vi "HP Loop.vi"(8 "error in (no error)":errorcluster, 11 "ValveControlModule in":refnum<class "DigitalControlModule.lvclass">) -> (0 "error out":errorcluster, 3 "ValveControlModule out":refnum<class "DigitalControlModule.lvclass">)   [LabVIEW 2023, in "VolatusControl.lvlib" / "DigitalControlModule.lvclass"]
uses:
  DigitalControlModule.lvclass
  DigitalControlModule.lvclass/DigitalControlModule.ctl
  <vilib>/Platform/TimedLoop/XDataNode/wakeup.ctl
  <vilib>/Platform/TimedLoop/XDataNode/XDNodeRunTimeDep.lvlib
  <vilib>/Platform/TimedLoop/XDataNode/nitl_modes.ctl
  <vilib>/Platform/TimedLoop/XDataNode/timing_clust.ctl
  <vilib>/platform/TimedLoop/XDataNode/XDataNode.xnode
  Volatus/Module/Module.lvclass
  C:/dev/volatus/mts-volatus-super/libs/lv-volatus/Volatus/Module/Module.lvclass
  C:/dev/volatus/mts-volatus-super/libs/lv-volatus/VolatusControl/DigitalControlModule/DigitalControlModule.lvclass
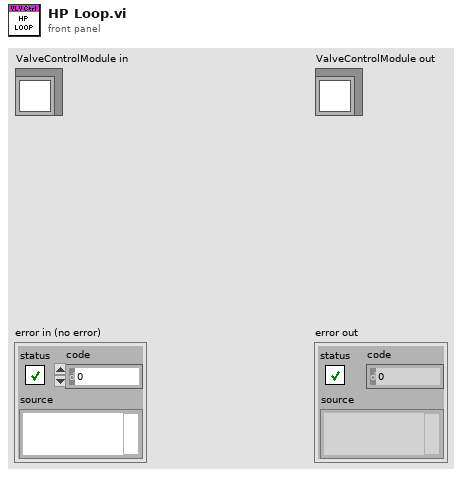
[diagram p1: front panel]
types:
  T1 = typedef "XDNodeRunTimeDep.lvlib/timing_clust.ctl" = cluster{"Expected End [f-1]":u64, "Actual End [f-1]":u64, "Finished Late? [f-1]":bool, "Expected End [i-1]":u64, "Actual End [i-1]":u64, "Finished Late? [i-1]":bool, "Expected Start [i]":u64, "Actual Start [i]":u64, "Expected Start [f]":u64, "Actual Start [f]":u64, "Source Name":string, "Structure Name":string, "Period":i64, "Deadline":i64, "Offset":i64, "Start":i64, "Priority":i32, "Timeout":i32, "Mode":T2, "Wakeup Reason":T3, "Error":errorcluster, "Source Type":string, "Secondary Source Type":string, "Global End Time":u64, "Global Start Time":u64, "Frame Duration":u64, "Iteration Duration":u64, "Assigned CPU":i32, "I/O Scan Engine Mode":u32}
  T2 = typedef "XDNodeRunTimeDep.lvlib/nitl_modes.ctl" = enum32{"No Change", "Process missed periods, maintain original phase", "Discard missed periods, maintain original phase", "Process missed periods, ignore original phase", "Discard missed periods, ignore original phase"}
  T3 = typedef "XDNodeRunTimeDep.lvlib/wakeup.ctl" = enum32{"Normal", "Aborted", "Asynchronous wakeup", "Timing source error", "Timed loop error", "Timeout"}
  T4 = enum32{"Invalid", "Standard", "Closed", "Hidden", "Minimized", "Maximized"}
  T5 = typedef "CmdDigitalMultiple.lvlib/Data.ctl" = cluster{"values":T6[]}
  T6 = typedef "CmdDigital.lvlib/Data.ctl" = cluster{"channel":string, "value":bool}
  T7 = typedef "CmdAnalogMultiple.lvlib/Data.ctl" = cluster{"values":T8[]}
  T8 = typedef "CmdAnalog.lvlib/Data.ctl" = cluster{"channel":string, "value":dbl}
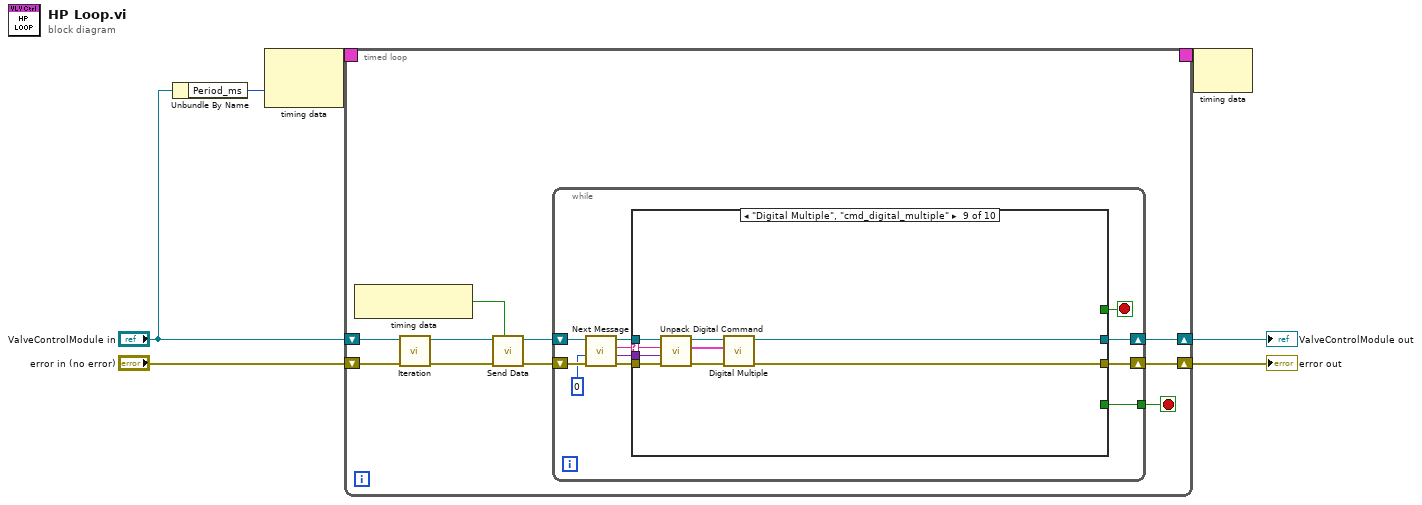
[diagram p0: block diagram]
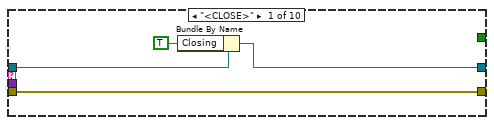
[diagram p2: hidden frame]
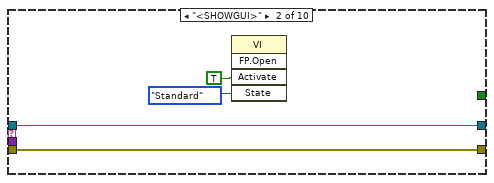
[diagram p3: hidden frame]
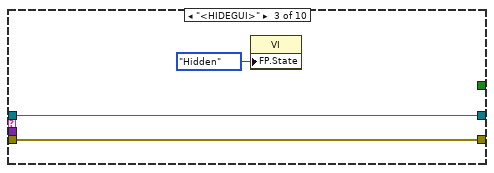
[diagram p4: hidden frame]
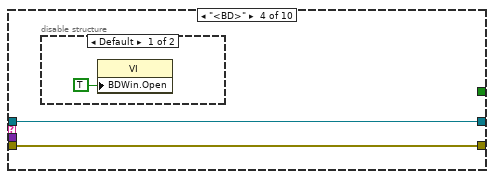
[diagram p5: hidden frame]
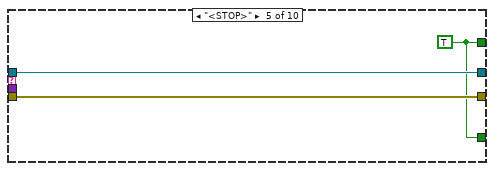
[diagram p7: hidden frame]
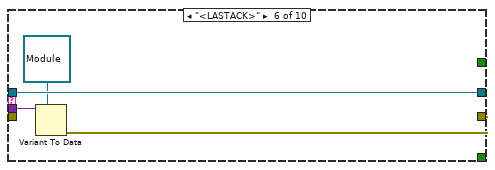
[diagram p8: hidden frame]
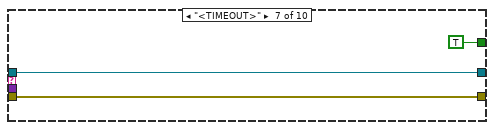
[diagram p9: hidden frame]
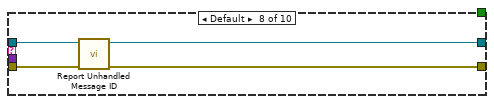
[diagram p10: hidden frame]
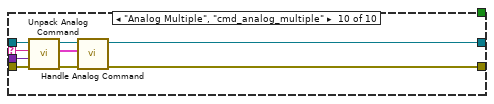
[diagram p11: hidden frame]
diagram:
  n1 = Unbundle By Name("ValveControlModule in") -> ("Period_ms"=w1:i64)
  n2 = node-c288(w1) -> (w7:T1)  [unwired: 1 in]
  n3 = timed-loop {
    shift-right: [w17] -> w4
    shift-left: "ValveControlModule in" -> [w12]
    shift-right: [w16] -> w3
    shift-left: "error in (no error)" -> [w11]
    timing: w7 -> [_]
    timing-out: [_] -> w6
    stop <- w15 stop-if-true
    n4 = node-c288() -> (w8:bool)  [unwired: 1 in]
    n5 = call "Iteration.vi"("error in (no error)"=w11, "ValveControlModule in"=w12) -> ("error out"=w13:errorcluster, "ValveControlModule out"=w14:refnum<class "DigitalControlModule.lvclass">)  [unwired: 8 in]
    n6 = call "Send Data.vi"("Finished Late"=w8, "error in (no error)"=w13, "ValveControlModule in"=w14) -> ("error out"=w10:errorcluster, "ValveControlModule out"=w9:refnum<class "DigitalControlModule.lvclass">)  [unwired: 7 in]
    n7 = while {
      tunnel: [w25] -> w15
      shift-right: [w26] -> w16
      shift-left: w10 -> [w23]
      shift-right: [w27] -> w17
      shift-left: w9 -> [w22]
      stop <- w20 stop-if-true
      n8 = call "Next Message.vi"("error in (no error)"=w23, "Timeout/Period ms (-1)"=0 ("Timeout ms (-1)"), "Module in"=w22) -> ("error out"=w30:errorcluster, "Data"=w24:variant, "ID"=w29:string, "Module out"=w28:refnum<class "DigitalControlModule.lvclass">)  [unwired: 5 in]
      n9 = case shown="\"Digital Multiple\", \"cmd_digital_multiple\"" w29 {
        selector: w29 -> [_ _ _ _ _ _ _ _ w63 w73]
        tunnel: w30 -> [w34 w37 w40 w42 w46 _ w53 w58 w61 w75]
        tunnel: w28 -> [w33 w38 w41 w43 w47 w51 w54 w56 w67 w76]
        tunnel: [w32 w38 w41 w43 w47 w51 w54 w55 w65 w69] -> w27
        tunnel: [w34 w37 w40 w42 w46 w48 w53 w57 w66 w68] -> w26
        tunnel: [_ _ _ _ w45 _ _ _ _ _] -> w25
        tunnel: w24 -> [_ _ _ _ _ w50 _ _ w62 w74]
        tunnel: [_ _ _ _ w45 _ TRUE _ _ _] -> w20
        frame "<CLOSE>" {
          n10 = Bundle By Name(cluster=w33, "Closing"=TRUE) -> (w32:refnum<class "DigitalControlModule.lvclass">)
        }
        frame "<SHOWGUI>" {
          n11 = invoke class="VI" method="FP.Open"("Activate"=TRUE ("Activate?"), "State"=T4."Standard") -> ()  [unwired: 3 in, 5 out]
        }
        frame "<HIDEGUI>" {
          n12 = property class="VI"("FP.State"=T4."Hidden" ("Front Panel Window:State")) -> ()  [unwired: 2 in, 2 out]
        }
        frame "<BD>" {
          n13 = disable-structure shown="Default" {
            frame condition #0 (active) {
              n14 = property class="VI"("BDWin.Open"=TRUE ("Block Diagram Window:Open")) -> ()  [unwired: 2 in, 2 out]
            }
            frame condition #1 {
            }
          }
        }
        frame "<STOP>" {
          w45 = TRUE
        }
        frame "<LASTACK>" {
          n15 = Variant To Data(type=refnum<class "Module.lvclass"> refnum ("Volatus:Module"), Variant=w50) -> (error out=w48:errorcluster)  [unwired: 1 in, 1 out]
        }
        frame "<TIMEOUT>" {
        }
        frame Default {
          n16 = call "Report Unhandled Message ID.vi"("error in (no error)"=w58, "Module in"=w56) -> ("error out"=w57:errorcluster, "Module out"=w55:refnum<class "DigitalControlModule.lvclass">)  [unwired: 8 in]
        }
        frame "Digital Multiple", "cmd_digital_multiple" {
          n17 = call "Unpack Digital Command.vi"("error in (no error)"=w61, "Data"=w62, "Type"=w63, "Module in"=w67) -> ("error out"=w60:errorcluster, "CmdDigitalMultiple"=w59:T5, "Module out"=w64:refnum<class "DigitalControlModule.lvclass">)  [unwired: 3 in, 2 out]
          n18 = call "Digital Multiple.vi"("error in (no error)"=w60, "Data"=w59, "ValveControlModule in"=w64) -> ("error out"=w66:errorcluster, "ValveControlModule out"=w65:refnum<class "DigitalControlModule.lvclass">)  [unwired: 7 in]
        }
        frame "Analog Multiple", "cmd_analog_multiple" {
          n19 = call "Unpack Analog Command.vi"("error in (no error)"=w75, "Data"=w74, "Type"=w73, "Module in"=w76) -> ("error out"=w70:errorcluster, "CmdAnalogMultiple"=w72:T7, "Module out"=w71:refnum<class "DigitalControlModule.lvclass">)  [unwired: 3 in, 2 out]
          n20 = call "Handle Analog Command.vi"("error in (no error)"=w70, "Command"=w72, "DigitalControlModule in"=w71) -> ("error out"=w68:errorcluster, "DigitalControlModule out"=w69:refnum<class "DigitalControlModule.lvclass">)  [unwired: 7 in]
        }
      }
    }
  }
  "error out" <- w3
  "ValveControlModule out" <- w4
  n21 = node-c288(w6) -> ()  [unwired: 1 out]
